vi "Get Product Name.vi"() -> (3 "Product Name":string="QC-X Thread Profiler")   [LabVIEW 2015, in "Tool Cfg.lvlib"]
uses:
  Tool Cfg.lvlib
  ConfigGLOB.vi
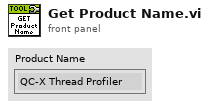
[diagram p1: front panel]
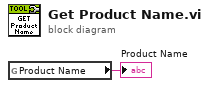
[diagram p0: block diagram]
diagram:
  n1 = global read "ConfigGLOB.vi" "Product Name"() -> (→"Product Name":string)
